vi "CLAD Exercise 3-6.vi"() -> ()   [LabVIEW 2014]
panel:
  in  "Kelvin":bool
  in  "Kevlin":bool
  out "Conversion":dbl
  out "Conversion":dbl
  in  "Tempature (C)":dbl
  in  "Tempature (F)":dbl
  # "Celsius"
  # "Fahrenheit"
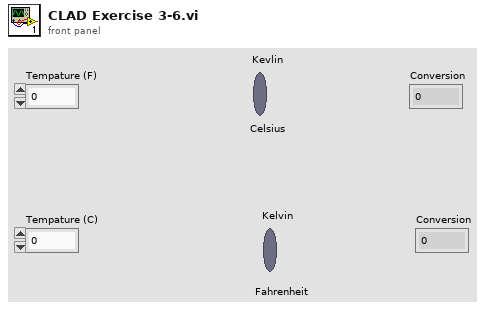
[diagram p1: front panel]
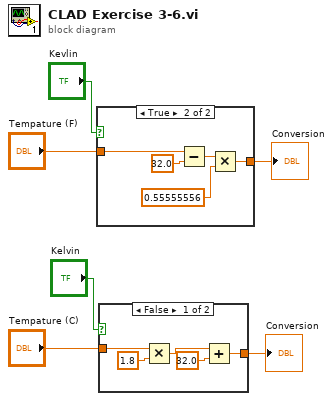
[diagram p0: block diagram]
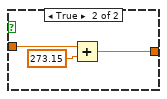
[diagram p2: hidden frame]
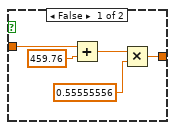
[diagram p3: hidden frame]
diagram:
  n1 = case shown="True" "Kevlin" {
    tunnel: "Tempature (F)" -> [w10 w16]
    tunnel: [w7 w12] -> w1
    frame False {
      n2 = Add(x=w10, y=459.76) -> (x+y=w9:dbl)
      n3 = Multiply(x=w9, y=0.55555556) -> (x*y=w7:dbl)
    }
    frame True {
      n4 = Subtract(x=w16, y=32.0) -> (x-y=w15:dbl)
      n5 = Multiply(x=w15, y=0.55555556) -> (x*y=w12:dbl)
    }
  }
  "Conversion" <- w1
  n6 = case shown="False" "Kelvin" {
    tunnel: "Tempature (C)" -> [w21 w24]
    tunnel: [w17 w22] -> w2
    frame False {
      n7 = Multiply(x=w21, y=1.8) -> (x*y=w19:dbl)
      n8 = Add(x=w19, y=32.0) -> (x+y=w17:dbl)
    }
    frame True {
      n9 = Add(x=w24, y=273.15) -> (x+y=w22:dbl)
    }
  }
  "Conversion" <- w2
